vi "PV ActiveLine - FullScaleRange (TPG362).vi"(7 "W/R":bool, 8 "Fehler (Eingang)":errorcluster, 9 "Sensor 2 Set":i8(ring)=3 items=["0.01 mbar", "0.1 mbar", "1 mbar", "10 mbar", "100 mbar", "1000 mbar", "2 bar", "5 bar", "10 bar", "50 bar"], 10 "Sensor 1 Set":i8(ring)=3 items=["0.01 mbar", "0.1 mbar", "1 mbar", "10 mbar", "100 mbar", "1000 mbar", "2 bar", "5 bar", "10 bar", "50 bar"], 11 "Referenz in":refnum<visa-resource-name>) -> (0 "Cluster (Ausgang)":errorcluster, 1 "Sensor 2 Get":i8(ring)=3 items=["0.01 mbar", "0.1 mbar", "1 mbar", "10 mbar", "100 mbar", "1000 mbar", "2 bar", "5 bar", "10 bar", "50 bar"], 2 "Sensor 1 Get":i8(ring)=3 items=["0.01 mbar", "0.1 mbar", "1 mbar", "10 mbar", "100 mbar", "1000 mbar", "2 bar", "5 bar", "10 bar", "50 bar"], 3 "Referenz out":refnum<visa-resource-name>)   [LabVIEW 2013, in "PV ActiveLine.lvlib"]
doc: "FSR - Measurement Range (F.S.) of Linear Gauges [hPa = mbar]\n\nTransmit: FSR [,a,b]\nReceive: a,b\n\nFull scale value gauge 1, \na =\n\n0 –> 0.01 hPa\n1 –> 0.1 hPa\n2 –> 1 hPa\n3 –> 10 hPa\n4 –> 100 hPa\n5 –> 1000 hPa (default)\n6 –> 200 kPa\n7 –> 500 kPa\n8 –> 1000 kPa\n9 –> 5000 kPa\n\nFull scale value gauge 2,\nb=\n\n0 –> 0.01 hPa\n1 –> 0.1 hPa\n2 –> 1 hPa\n3 –> 10 hPa\n4 –> 100 hPa\n5 –> 1000 hPa (default)\n6 –> 200 kPa\n7 –> 500 kPa\n8 –> 1000 kPa\n9 –> 5000 kPa"
uses:
  C:/Program Files (x86)/National Instruments/LabVIEW 2013/PV ActiveLine/PV ActiveLine.lvlib
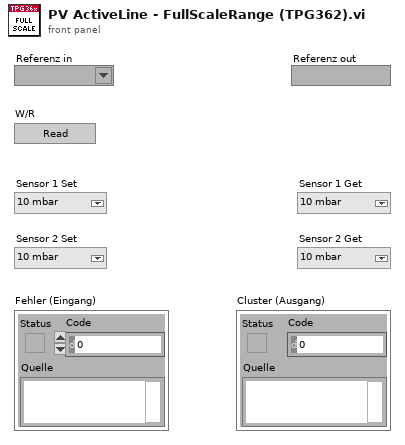
[diagram p1: front panel]
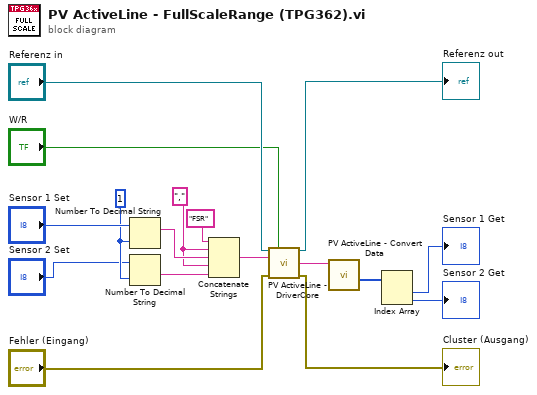
[diagram p0: block diagram]
diagram:
  w10 = ","
  w6 = i16 1 ("width (-)")
  n1 = Number To Decimal String(number="Sensor 1 Set", width (-)=w6) -> (decimal integer string=w12:string)
  n2 = Number To Decimal String(number="Sensor 2 Set", width (-)=w6) -> (decimal integer string=w11:string)
  n3 = Concatenate Strings("FSR", w10, w12, w10, w11) -> (w9:string)
  n4 = call "PV ActiveLine - DriverCore.vi"("Referenz in"="Referenz in", "Write/Read"="W/R", "Command"=w9, "Fehler (Eingang)"="Fehler (Eingang)") -> ("Referenz out"=→"Referenz out":refnum<visa-resource-name>, "String Out"=w4:string, "Cluster (Ausgang)"=→"Cluster (Ausgang)":errorcluster)  [unwired: 9 in]
  n5 = call "PV ActiveLine - Convert Data.vi"("String in"=w4) -> ("Integer Out"=w3:i32[])  [unwired: 7 in, 3 out]
  n6 = Index Array(array=w3) -> (element #1=→"Sensor 1 Get":i32, element #2=→"Sensor 2 Get":i32)  [unwired: 2 in]
